vi "Build.vi"(6 "Assembly Type":string, 8 "Position":i32, 9 "XYZTheta":dbl[](array[numeric]), 10 "text file":dbl[][](array[numeric]), 11 "Sensor Dispense in":refnum<class "Sensor Dispense.lvclass">) -> (3 "Sensor Dispense out":refnum<class "Sensor Dispense.lvclass">)   [LabVIEW 2021, in "Sensor Dispense.lvclass"]
uses:
  Projects/Sensor Dispense.lvclass
  C:/Users/HEP/Documents/GitHub/Gantry/UCSB-Gantry-HEP-main/Classes/Routine/Dispense/Dispense.lvclass
  Projects/Sensor Dispense.lvclass/Sensor Dispense.ctl
  <vilib>/Analysis/coordinate.llb/2D Cartesian Coordinate Rotation (Scalar).vi
  <vilib>/Analysis/NI_AALPro.lvlib
panel:
  out "CW/CCW":dbl[](array[numeric])
  out "CW/CCW":dbl[](array[numeric])
  out "endpoints 2":dbl[][](array[numeric])
  out "endpoints":dbl[][](array[numeric])
  out "data":T1(array[cluster])
  out "cell count":dbl[](array[numeric])
  out "centers":dbl[][](array[numeric])
  # "[x1,y1,x2,y2]"
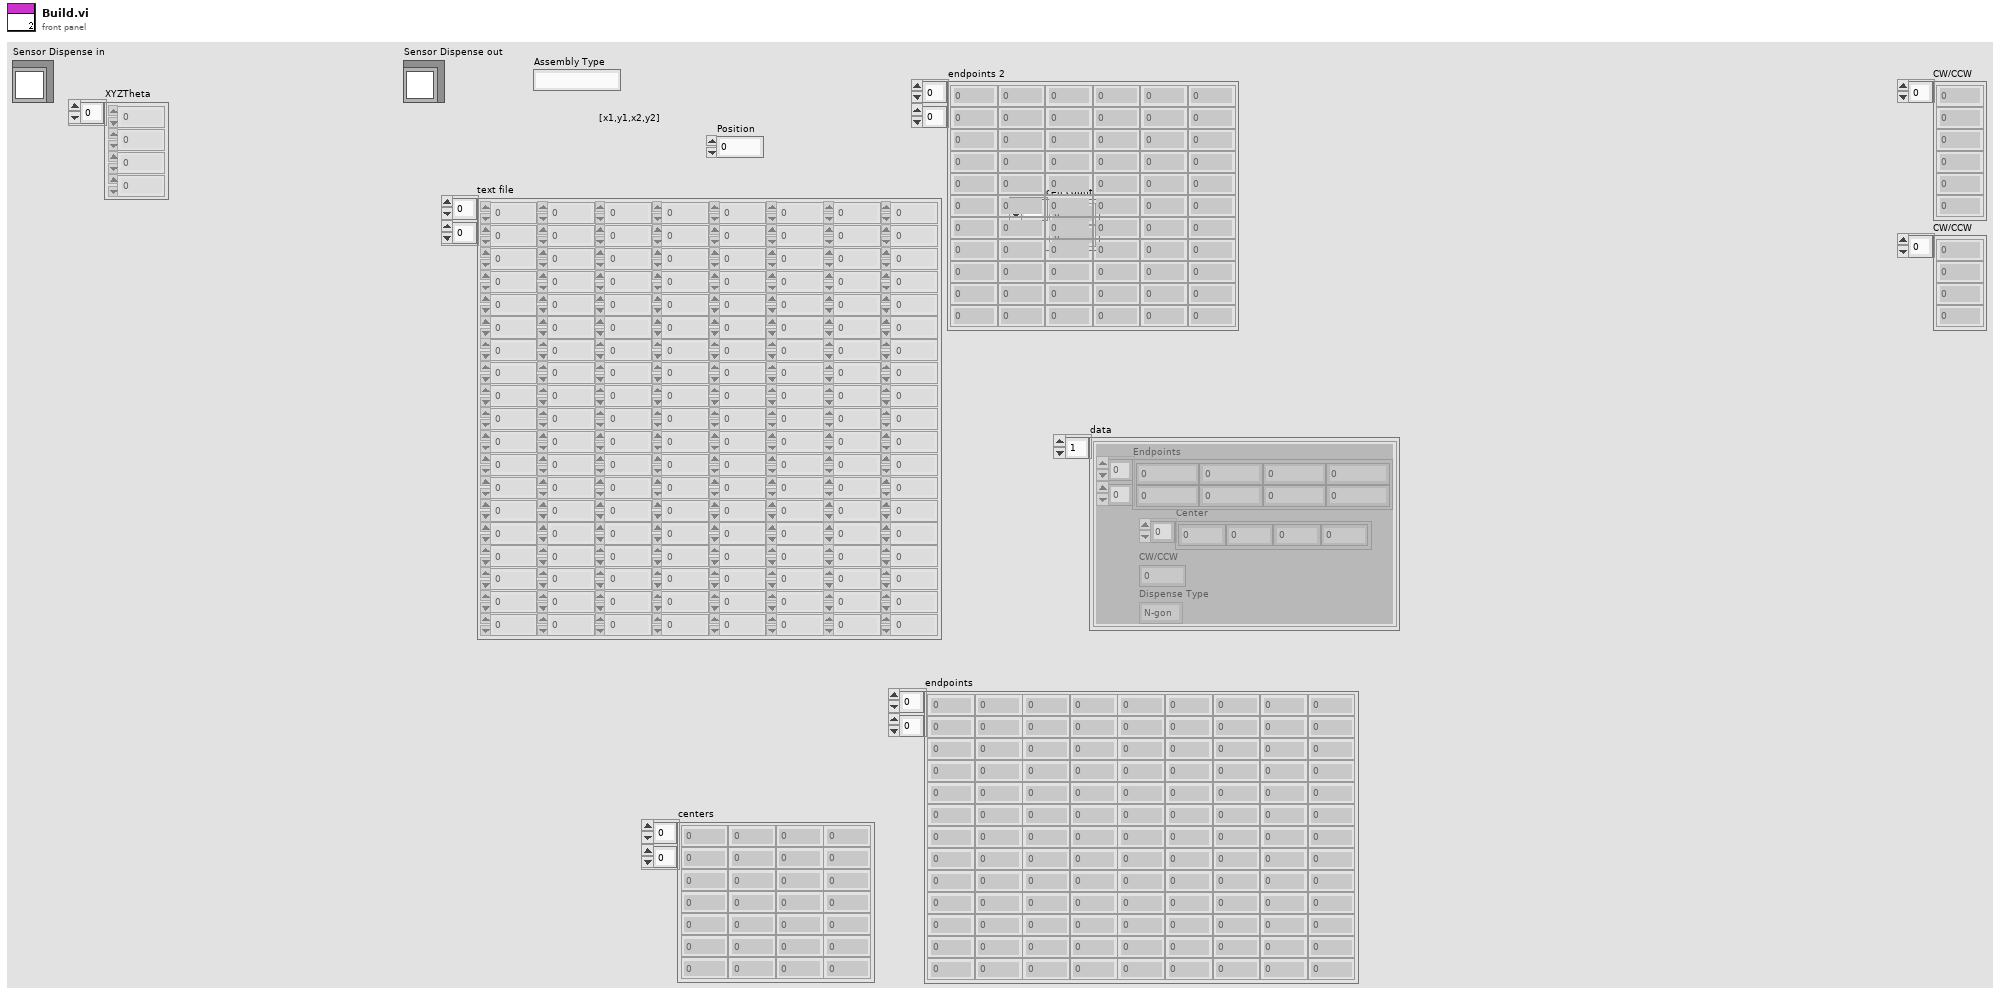
[diagram p1: front panel]
types:
  T1 = cluster{"Endpoints":dbl[][], "Center":dbl[], "CW/CCW":dbl, "Dispense Type":enum16{"N-gon", "Square", "Arc", "Dot", "Line", "Circle"}}[]
  T2 = enum16{"N-gon", "Square", "Arc", "Dot", "Line", "Circle"}
  T3 = cluster{"Endpoints":dbl[][], "Center":dbl[], "CW/CCW":dbl, "Dispense Type":enum16{"N-gon", "Square", "Arc", "Dot", "Line", "Circle"}}
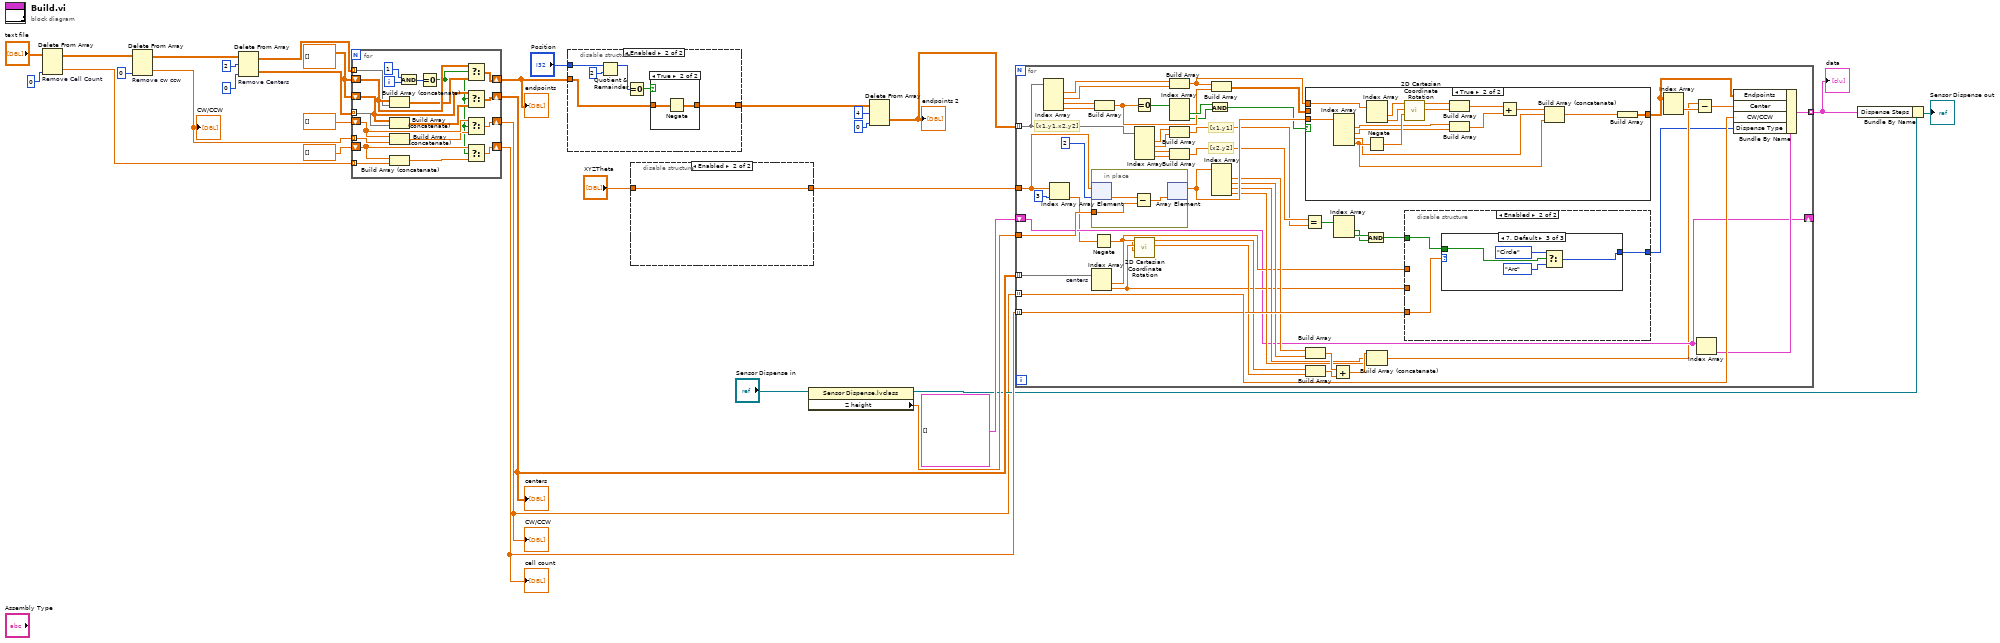
[diagram p0: block diagram]
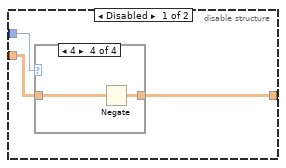
[diagram p2: hidden frame]
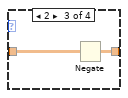
[diagram p5: hidden frame]
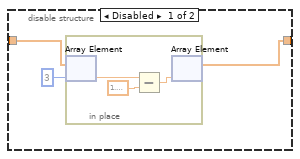
[diagram p7: hidden frame]
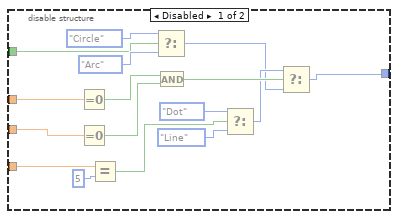
[diagram p8: hidden frame]
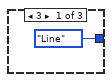
[diagram p9: hidden frame]
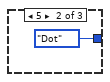
[diagram p10: hidden frame]
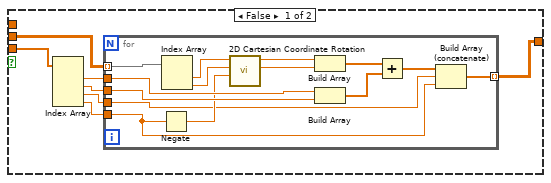
[diagram p11: hidden frame]
diagram:
  w28 = dbl[][] []
  n1 = Delete From Array "Remove Cell Count"(array="text file", index (col)=0) -> (deleted portion=w22:dbl[], array with subset deleted=w24:dbl[][])  [unwired: 2 in]
  n2 = Delete From Array "Remove cw ccw"(array=w24, index (col)=0 ("disabled index (col)")) -> (deleted portion=w5:dbl[], array with subset deleted=w21:dbl[][])  [unwired: 2 in]
  "CW/CCW" <- w5
  n3 = Delete From Array "Remove Centers"(array=w21, length=2, index (col)=0) -> (deleted portion=w17:dbl[][], array with subset deleted=w18:dbl[][])  [unwired: 1 in]
  n4 = for {
    tunnel: w18 -> [w47] mode=indexing
    shift-right: [w45] -> w2
    shift-left: w28 -> [w48]
    tunnel: w17 -> [w44] mode=indexing
    shift-right: [w41] -> w29
    shift-left: w28 -> [w42]
    tunnel: w22 -> [w40] mode=indexing
    shift-right: [w37] -> w26
    shift-left: dbl[] [] -> [w39]
    shift-right: [w32] -> w4
    shift-left: dbl[] [] -> [w35]
    tunnel: w5 -> [w36] mode=indexing
    i -> [w50]
    n5 = Build Array (concatenate)(w48, w47) -> (w46:dbl[][])
    n6 = Build Array (concatenate)(w42, w44) -> (w43:dbl[][])
    n7 = Build Array (concatenate)(w35, w36) -> (w34:dbl[])
    n8 = Build Array (concatenate)(w39, w40) -> (w38:dbl[])
    n9 = And(x=1, y=w50) -> (x .and. y?=w49:i32)
    n10 = Equal To 0?(x=w49) -> (x = 0?=w33:bool)
    n11 = Select(t=w48, s=w33, f=w46) -> (s? t:f=w45:dbl[][])
    n12 = Select(t=w42, s=w33, f=w43) -> (s? t:f=w41:dbl[][])
    n13 = Select(t=w35, s=w33, f=w34) -> (s? t:f=w32:dbl[])
    n14 = Select(t=w39, s=w33, f=w38) -> (s? t:f=w37:dbl[])
  }
  "centers" <- w29
  "cell count" <- w26
  "endpoints" <- w2
  "CW/CCW" <- w4
  n15 = disable-structure shown="Enabled" {
    disable-tunnel: "Position" -> [w54 w66]
    disable-tunnel: [w53 w61] -> w3
    disable-tunnel: w2 -> [w52 w62]
    frame Disabled {
      n16 = case shown="4" w54 {
        tunnel: [w55 w56 w58 w60] -> w53
        tunnel: w52 -> [w55 w56 w57 w59]
        frame 1, Default {
        }
        frame 3 {
        }
        frame 2 {
          n17 = Negate(x=w57) -> (-x=w58:dbl[][])
        }
        frame 4 {
          n18 = Negate(x=w59) -> (-x=w60:dbl[][])
        }
      }
    }
    frame Enabled {
      n19 = Quotient & Remainder(x=w66, y=2) -> (x-y*floor(x/y)=w64:i32)  [unwired: 1 out]
      n20 = Equal To 0?(x=w64) -> (x = 0?=w63:bool)
      n21 = case shown="True" w63 {
        tunnel: w62 -> [w67 w69]
        tunnel: [w67 w68] -> w61
        frame False {
        }
        frame True {
          n22 = Negate(x=w69) -> (-x=w68:dbl[][])
        }
      }
    }
  }
  n23 = disable-structure shown="Enabled" {
    disable-tunnel: "XYZTheta" -> [w72 w76]
    disable-tunnel: [w70 w76] -> w7
    frame Disabled {
      n24 = in-place {
        n25 = in-place-array #1(w72, 3) -> (w75:dbl)
        n26 = Subtract(x=w75, y=1.5707963267948966) -> (x-y=w73:dbl)
        n27 = in-place-array #1(w73) -> (w70:dbl[])  [unwired: 1 out]
      }
    }
    frame Enabled {
    }
  }
  n28 = property class="Sensor Dispense.lvclass"(reference="Sensor Dispense in") -> (reference out=w14:refnum<class "Sensor Dispense.lvclass">, "Z height"=w31:dbl)  [unwired: 1 in, 1 out]
  n29 = Delete From Array(array=w3, length=4, index (col)=0 ("disabled index (col)")) -> (deleted portion=w9:dbl[][])  [unwired: 1 in, 1 out]
  "endpoints 2" <- w9
  n30 = for {
    tunnel: w9 -> [w91] mode=indexing
    tunnel: w7 -> [w100]
    tunnel: w31 -> [w127]
    tunnel: w29 -> [w126] mode=indexing
    tunnel: w4 -> [w125] mode=indexing
    tunnel: w26 -> [w124] mode=indexing
    shift-right: [w109] -> _
    shift-left: T1 [] ("Dispense Steps") -> [w109]
    tunnel: [w123] -> w13 mode=indexing
    # "[x2,y2]"
    # "[x1,y1]"
    # "[x1,y1,x2,y2]"
    n31 = Index Array(array=w91) -> (element #1=w89:dbl, element #2=w88:dbl, element #3=w87:dbl, element #4=w86:dbl)  [unwired: 4 in]
    n32 = Index Array(array=w100, index=3) -> (element=w99:dbl)
    n33 = in-place {
      in-place-border: w127 -> [w154]
      n34 = in-place-array #2(w100, 2) -> (w155:dbl)
      n35 = Subtract(x=w155, y=w154) -> (x-y=w153:dbl)
      n36 = in-place-array #2(w153) -> (w120:dbl[])  [unwired: 1 out]
    }
    n37 = Index Array "centers"(array=w126) -> (element #1=w112:dbl, element #2=w111:dbl)  [unwired: 2 in]
    n38 = Negate(x=w99) -> (-x=w98:dbl)
    n39 = Build Array(w87, w86) -> (w83:dbl[])
    n40 = Equal To 0?(x=w83) -> (x = 0?=w82:bool[])
    n41 = Index Array(array=w91) -> (element #1=w96:dbl, element #2=w95:dbl, element #3=w108:dbl, element #4=w107:dbl)  [unwired: 4 in]
    n42 = call-poly <vilib>:"2D Cartesian Coordinate Rotation.vi"("theta"=w98, "y"=w111, "x"=w112) -> ("y out"=w121:dbl, "x out"=w122:dbl)  [unwired: 6 in, 1 out]
    n43 = Build Array(w89, w88) -> (w79:dbl[])
    n44 = Index Array(array=w82) -> (element #1=w84:bool, element #2=w80:bool)  [unwired: 2 in]
    n45 = Build Array(w96, w95) -> (w105:dbl[])
    n46 = Build Array(w108, w107) -> (w106:dbl[])
    n47 = And(x=w84, y=w80) -> (x .and. y?=w81:bool)
    n48 = Build Array(w79, w83) -> (w85:dbl[][])
    n49 = Index Array(array=w120) -> (element #1=w119:dbl, element #2=w116:dbl, element #3=w114:dbl, element #4=w113:dbl)  [unwired: 4 in]
    n50 = Equal?(x=w106, y=w105) -> (x = y?=w104:bool[])
    n51 = case shown="True" w81 {
      tunnel: w120 -> [w162 w189]
      tunnel: [w161 w177] -> w77
      tunnel: w85 -> [w160 _]
      tunnel: w79 -> [_ w192]
      frame False {
        n52 = Index Array(array=w162) -> (element #1=w159:dbl, element #2=w158:dbl, element #3=w156:dbl, element #4=w157:dbl)  [unwired: 4 in]
        n53 = for {
          tunnel: w160 -> [w176] mode=indexing
          tunnel: w159 -> [w173]
          tunnel: w158 -> [w172]
          tunnel: [w163] -> w161 mode=indexing
          tunnel: w157 -> [w164]
          tunnel: w156 -> [w165]
          n54 = Negate(x=w164) -> (-x=w167:dbl)
          n55 = Index Array(array=w176) -> (element #1=w175:dbl, element #2=w174:dbl)  [unwired: 2 in]
          n56 = call-poly <vilib>:"2D Cartesian Coordinate Rotation.vi"("theta"=w167, "y"=w174, "x"=w175) -> ("y out"=w170:dbl, "x out"=w171:dbl)  [unwired: 6 in, 1 out]
          n57 = Build Array(w171, w170) -> (w169:dbl[])
          n58 = Build Array(w173, w172) -> (w168:dbl[])
          n59 = Add(x=w169, y=w168) -> (x+y=w166:dbl[])
          n60 = Build Array (concatenate)(w166, w165, w164) -> (w163:dbl[])
        }
      }
      frame True {
        n61 = Index Array(array=w189) -> (element #1=w185:dbl, element #2=w184:dbl, element #3=w180:dbl, element #4=w181:dbl)  [unwired: 4 in]
        n62 = Negate(x=w181) -> (-x=w188:dbl)
        n63 = Index Array(array=w192) -> (element #1=w191:dbl, element #2=w190:dbl)  [unwired: 2 in]
        n64 = call-poly <vilib>:"2D Cartesian Coordinate Rotation.vi"("theta"=w188, "y"=w190, "x"=w191) -> ("y out"=w186:dbl, "x out"=w187:dbl)  [unwired: 6 in, 1 out]
        n65 = Build Array(w187, w186) -> (w182:dbl[])
        n66 = Build Array(w185, w184) -> (w183:dbl[])
        n67 = Add(x=w182, y=w183) -> (x+y=w179:dbl[])
        n68 = Build Array (concatenate)(w179, w180, w181) -> (w178:dbl[])
        n69 = Build Array(w178) -> (w177:dbl[][])
      }
    }
    n70 = Build Array(w119, w116) -> (w118:dbl[])
    n71 = Build Array(w122, w121) -> (w117:dbl[])
    n72 = Add(x=w118, y=w117) -> (x+y=w115:dbl[])
    n73 = Index Array(array=w104) -> (element #1=w102:bool, element #2=w103:bool)  [unwired: 2 in]
    n74 = And(x=w103, y=w102) -> (x .and. y?=w101:bool)
    n75 = Build Array (concatenate)(w115, w114, w113) -> (w93:dbl[])
    n76 = disable-structure shown="Enabled" {
      disable-tunnel: w124 -> [w143 w146]
      disable-tunnel: w112 -> [w140 _]
      disable-tunnel: w111 -> [w139 _]
      disable-tunnel: w101 -> [w132 w145]
      disable-tunnel: [w128 w144] -> w90
      frame Disabled {
        n77 = Equal To 0?(x=w140) -> (x = 0?=w141:bool)
        n78 = Equal To 0?(x=w139) -> (x = 0?=w142:bool)
        n79 = Equal?(x=w143, y=5) -> (x = y?=w135:bool)
        n80 = Select(t=T2."Circle" ("Dispense Type"), s=w132, f=T2."Arc" ("Dispense Type")) -> (s? t:f=w129:T2)
        n81 = And(x=w141, y=w142) -> (x .and. y?=w131:bool)
        n82 = Select(t=T2."Dot" ("Dispense Type"), s=w135, f=T2."Line" ("Dispense Type")) -> (s? t:f=w130:T2)
        n83 = Select(t=w130, s=w131, f=w129) -> (s? t:f=w128:T2)
      }
      frame Enabled {
        n84 = case shown="7, Default" w146 {
          tunnel: w145 -> [_ _ w150]
          tunnel: [T2."Line" ("Dispense Type") T2."Dot" ("Dispense Type") w149] -> w144
          frame 3 {
          }
          frame 5 {
          }
          frame 7, Default {
            n85 = Select(t=T2."Circle" ("Dispense Type"), s=w150, f=T2."Arc" ("Dispense Type")) -> (s? t:f=w149:T2)
          }
        }
      }
    }
    n86 = Index Array(array=w77) -> (element=w94:dbl[])  [unwired: 2 in]
    n87 = Subtract(x=w93, y=w94) -> (x-y=w92:dbl[])
    n88 = Index Array(array=w109) -> (element=w110:T3)  [unwired: 1 in]
    n89 = Bundle By Name(cluster=w110, "Endpoints"=w77, "Center"=w92, "CW/CCW"=w125, "Dispense Type"=w90) -> (w123:T3)
  }
  "data" <- w13
  n90 = Bundle By Name(cluster=w14, "Dispense Steps"=w13) -> (→"Sensor Dispense out":refnum<class "Sensor Dispense.lvclass">)
